vi "Serial port communication (subVI).vi"() -> ()   [LabVIEW 2016]
doc: "This example performs a serial port write and a serial port read. The parameters set for the serial port must match the parameters of the connected instrument or device. The VISA Configure Serial Port VI sets the configuration parameters. The front panel displays the controls used to configure the basic parameters, such as baud rate, data bits, and parity. The VI passes the VISA resource name to other VIs that perform operations on that VISA resource. The VISA Write function sends a command to the serial device and the VISA Read function returns data based on the command. The VISA Close function then closes the reference to the serial device. It is important to close the reference; otherwise, further communication through that port might not be possible."
uses:
  C:/Program Files/National Instruments/LabVIEW 2015/examples/Instrument IO/Serial/support/Serial - Settings.ctl
  <vilib>/Instr/_visa.llb/VISA Configure Serial Port (Instr).vi
panel:
  in  "VISA resource name in":refnum<visa-resource-name>
  in  "Command (RT, RS..)":string(combo)="R"
  out "bytes read":u32
  in  "delay before read (ms)":u32=800
  out "Response":string
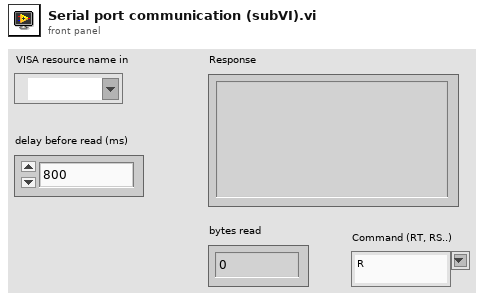
[diagram p1: front panel]
types:
  T1 = typedef "Serial - Settings.ctl" = cluster{"baud rate":u32, "data bits":u16, "parity":enum16{"None", "Odd", "Even", "Mark", "Space"}, "stop bits":u16, "flow control":u16}
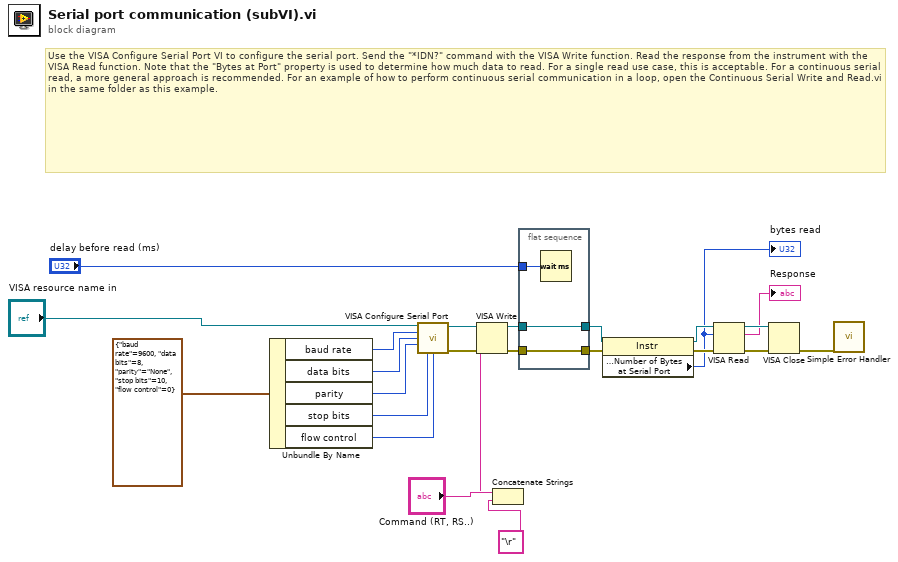
[diagram p0: block diagram]
diagram:
  # "Use the VISA Configure Serial Port VI to configure the serial port. Send the \"*IDN?\" command with the VISA Write function. Read the response from the instrument with the VISA Read function. Note that the \"Bytes at Port\" property is used to determine how much data to read. For a single read use case, this is acceptable. For a continuous serial read, a more general approach is recommended. For an example of how to perform continuous serial communication in a loop, open the Continuous Serial Write and Read.vi in the same folder as this example."
  n1 = Unbundle By Name(T1 {"baud rate"=9600, "data bits"=8, "parity"=enum."None", "stop bits"=10, "flow control"=0} ("Serial Settings")) -> ("baud rate"=w9:u32, "data bits"=w8:u16, "parity"=w7:enum16{"None", "Odd", "Even", "Mark", "Space"}, "stop bits"=w6:u16, "flow control"=w5:u16)
  n2 = call-poly "VISA Configure Serial Port"("VISA resource name"="VISA resource name in", "baud rate (9600)"=w9, "data bits (8)"=w8, "parity (0:none)"=w7, "stop bits (10: 1 bit)"=w6, "flow control (0:none)"=w5) -> ("VISA resource name out"=w23:refnum<visa-resource-name>, "error out"=w24:errorcluster)  [unwired: 3 in, 5 out]
  n3 = Concatenate Strings("Command (RT, RS..)", "\r" ("Command (RT\\r, RS\\r)")) -> (w2:string)
  n4 = VISA Write(VISA resource name=w23, write buffer=w2, error in (no error)=w24) -> (VISA resource name out=w17:refnum<visa-resource-name>, error out=w19:errorcluster)  [unwired: 1 out]
  n5 = flat-sequence {
    tunnel: w19 -> [w26]
    tunnel: [w26] -> w18
    tunnel: w17 -> [w25]
    tunnel: [w25] -> w16
    tunnel: "delay before read (ms)" -> [w27]
    frame #0 {
      n6 = Wait (ms)(milliseconds to wait=w27) -> ()  [unwired: 1 out]
    }
  }
  n7 = property class="Instr"(reference=w16, error in=w18) -> (reference out=w14:refnum<visa-resource-name>, error out=w13:errorcluster, "Serial Settings:Number of Bytes at Serial Port"=w11:u32)
  "bytes read" <- w11
  n8 = VISA Read(VISA resource name=w14, byte count=w11, error in (no error)=w13) -> (VISA resource name out=w21:refnum<visa-resource-name>, read buffer=→"Response":string, error out=w22:errorcluster)  [unwired: 1 out]
  n9 = VISA Close(VISA resource name=w21, error in (no error)=w22) -> (error out=w20:errorcluster)
  n10 = call <vilib>:"Simple Error Handler.vi"("error in (no error)"=w20) -> ()  [unwired: 1 in, 8 out]
